vi "AutoDrive PID.vi"(8 "Steady Val (no PID only)":dbl, 9 "Distance to travel (inches)":dbl, 10 "Desired RPM (PID only)":dbl, 11 "Use PID":bool) -> ()   [LabVIEW 2012]
uses:
  State_Machine_Enum.ctl
  Robot Global Data.vi
  <vilib>/addons/control/pid/pid.llb/PID (DBL).vi
  <vilib>/addons/control/pid/NI_PID_pid.lvlib
panel:
  in  "output range LEFT":cluster{"output high":dbl, "output low":dbl}={"output high"=1.0, "output low"=-1.0} {"output low" format="%.2f"; "output high" format="%.2f"}
  in  "Left PID Gains":T1={"proportional gain (Kc)"=0.015, "integral time (Ti, min)"=0.001, "derivative time (Td, min)"=0.0} {"derivative time (Td, min)" format="%.3f"; "integral time (Ti, min)" format="%.3f"; "proportional gain (Kc)" format="%.3f"}
  in  "output range RIGHT":cluster{"output high":dbl, "output low":dbl}={"output high"=1.0, "output low"=-1.0} {"output low" format="%.2f"; "output high" format="%.2f"}
  in  "Right PID Gains":T1={"proportional gain (Kc)"=0.015, "integral time (Ti, min)"=0.001, "derivative time (Td, min)"=0.0} {"derivative time (Td, min)" format="%.3f"; "integral time (Ti, min)" format="%.3f"; "proportional gain (Kc)" format="%.3f"}
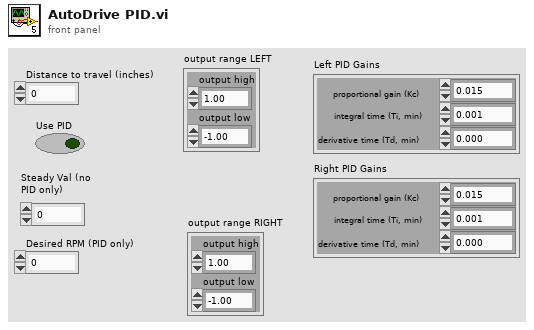
[diagram p1: front panel]
types:
  T1 = cluster{"proportional gain (Kc)":dbl, "integral time (Ti, min)":dbl, "derivative time (Td, min)":dbl}
  T2 = typedef "State_Machine_Enum.ctl" = enum16{"Idle", "Start", "Do", "Stop", "Init"}
  T3 = typedef "LoopDisable.ctl" = cluster{"Climb.vi":bool, "LauncherAngle.vi":bool, "Launcher.vi":bool, "ArmControl.vi":bool, "WinchMotor.vi":bool, "ReadDriveEncoder.vi":bool}
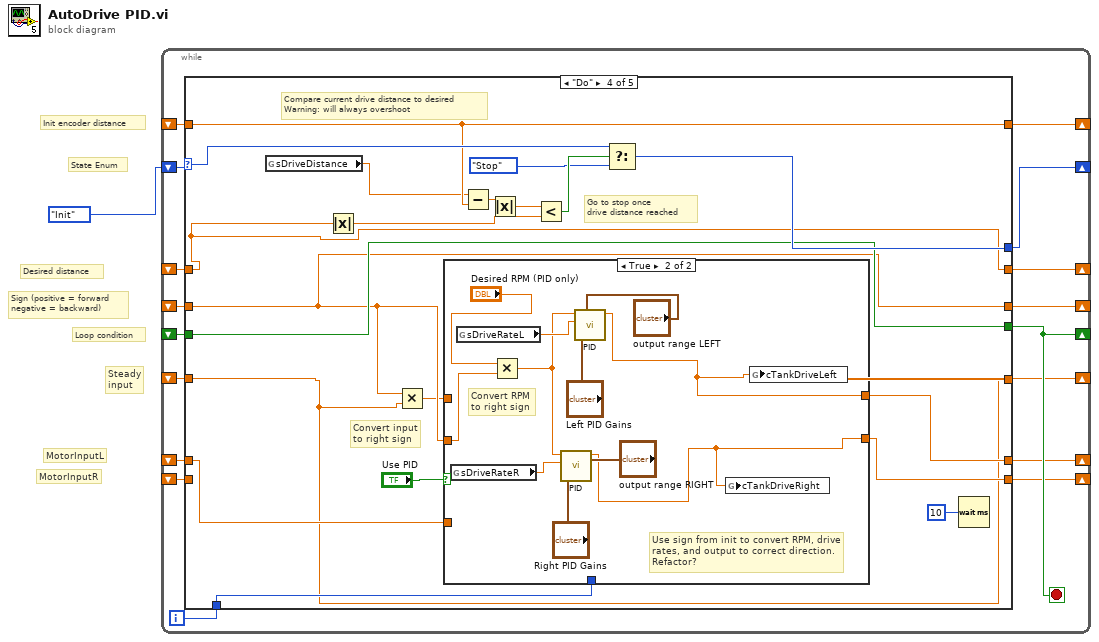
[diagram p0: block diagram]
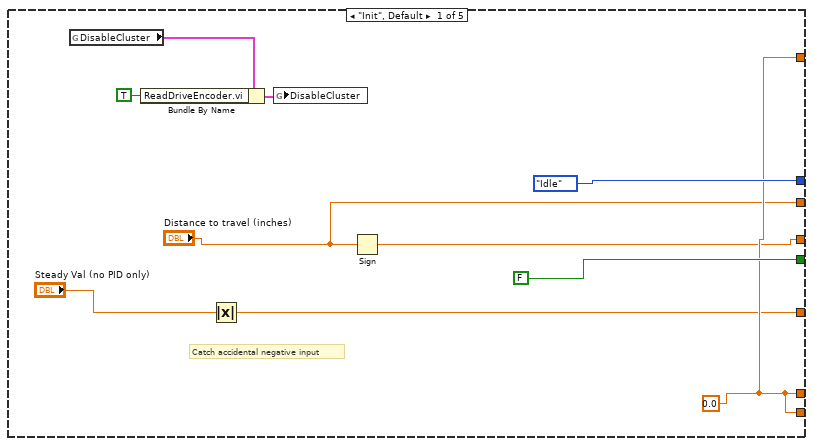
[diagram p2: hidden frame]
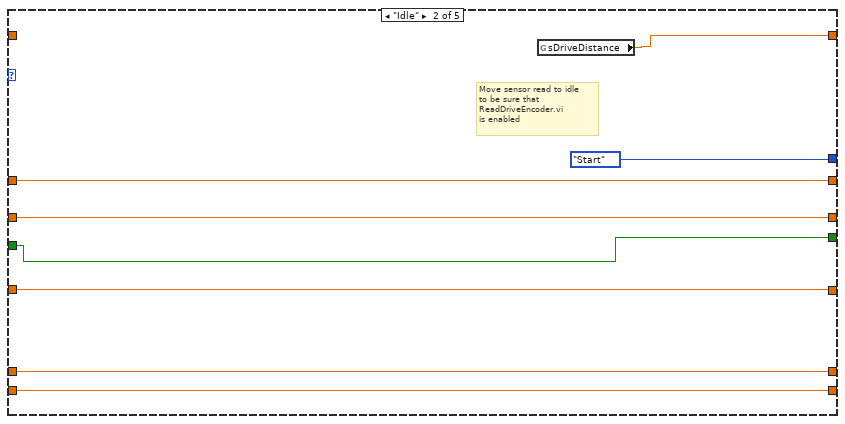
[diagram p3: hidden frame]
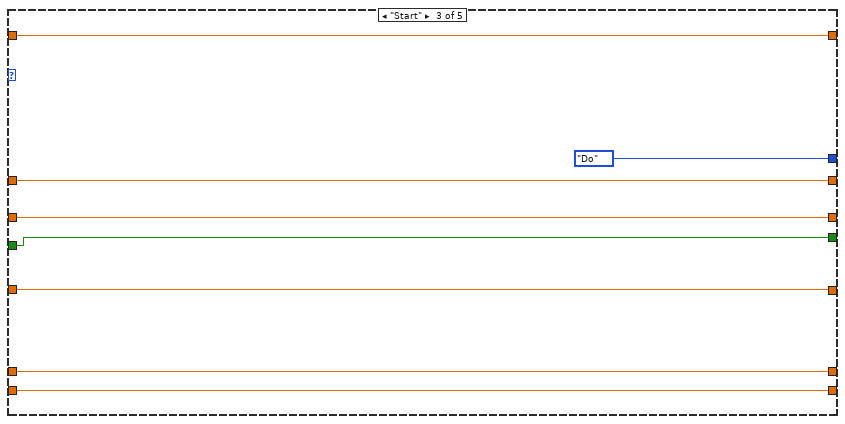
[diagram p4: hidden frame]
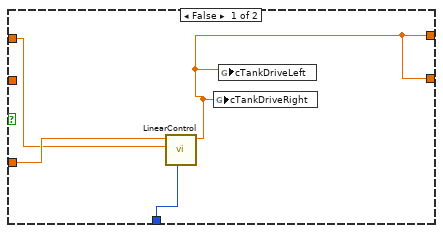
[diagram p5: hidden frame]
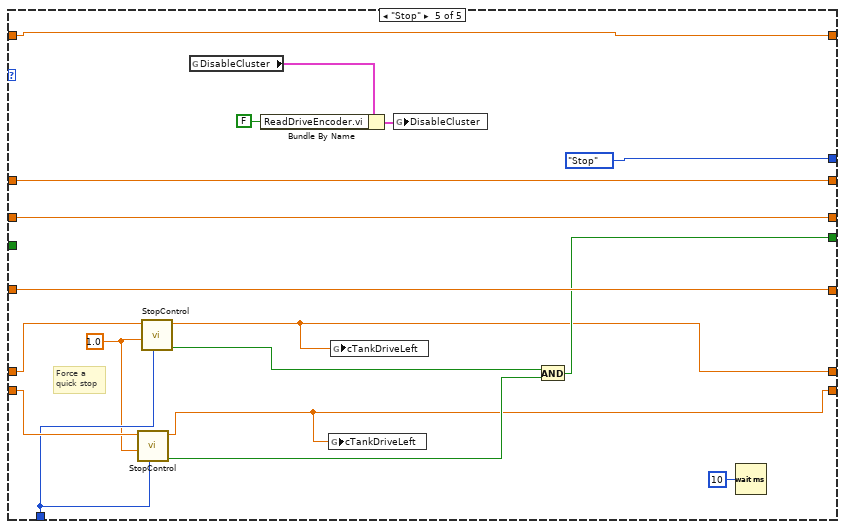
[diagram p6: hidden frame]
diagram:
  # "Desired distance"
  # "MotorInputR"
  # "MotorInputL"
  # "Sign (positive = forward\nnegative = backward)"
  # "Init encoder distance"
  # "State Enum"
  # "Loop condition"
  # "Steady\ninput"
  n1 = while {
    shift-right: [w17] -> _
    shift-left: State_Machine_Enum."Init" ("State") -> [w18]
    shift-right: [w16] -> _
    shift-left: _ -> [w15]
    shift-right: [w14] -> _
    shift-left: _ -> [w13]
    shift-right: [w12] -> _
    shift-left: _ -> [w11]
    shift-right: [w9] -> _
    shift-left: _ -> [w7]
    shift-right: [w10] -> _
    shift-left: _ -> [w8]
    shift-right: [w6] -> _
    shift-left: _ -> [w5]
    shift-right: [w3] -> _
    shift-left: _ -> [w2]
    i -> [w4]
    stop <- w16 stop-if-true
    n2 = case shown="\"Do\"" w18 {
      selector: w18 -> [_ _ _ w64 _]
      tunnel: [State_Machine_Enum."Idle" ("State") State_Machine_Enum."Start" ("State") State_Machine_Enum."Do" ("State") w63 State_Machine_Enum."Stop" ("State")] -> w17
      tunnel: [w19 w32 w40 w46 w88] -> w6
      tunnel: [FALSE w36 w44 w60 w85] -> w16
      tunnel: w15 -> [_ w36 w44 w60 _]
      tunnel: [w23 w31 w43 w58 w97] -> w14
      tunnel: w13 -> [_ _ w43 w58 w97]
      tunnel: [w21 w29 w41 w47 w95] -> w12
      tunnel: w11 -> [_ w29 w41 w47 w95]
      tunnel: [w23 w34 w39 w52 w83] -> w10
      tunnel: [w23 w33 w38 w51 w82] -> w9
      tunnel: w8 -> [_ w34 w39 w50 w90]
      tunnel: w7 -> [_ w33 w38 _ w89]
      tunnel: w5 -> [_ w32 w40 w46 w88]
      tunnel: w4 -> [_ _ _ w49 w81]
      tunnel: ["Distance to travel (inches)" w30 w37 w48 w84] -> w3
      tunnel: w2 -> [_ w30 w37 w48 w84]
      frame "Init", Default {
        w23 = 0.0 ("New Motor Input")
        # "Catch accidental negative input"
        n3 = global read "Robot Global Data.vi" "DisableCluster"() -> (w26:T3)
        n4 = Bundle By Name(cluster=w26, "ReadDriveEncoder.vi"=TRUE) -> (w25:T3)
        n5 = Absolute Value(x="Steady Val (no PID only)") -> (abs(x)=w19:dbl)
        n6 = global write "Robot Global Data.vi" "DisableCluster"(w25) -> ()
        n7 = Sign(1:"Distance to travel (inches)") -> (0:w21:dbl)
      }
      frame "Idle" {
        # "Move sensor read to idle\nto be sure that \nReadDriveEncoder.vi\nis enabled"
        n8 = global read "Robot Global Data.vi" "sDriveDistance"() -> (w31:dbl)
      }
      frame "Start" {
      }
      frame "Do" {
        # "Go to stop once\ndrive distance reached"
        # "Convert input\nto right sign"
        # "Compare current drive distance to desired\nWarning: will always overshoot"
        n9 = global read "Robot Global Data.vi" "sDriveDistance"() -> (w54:dbl)
        n10 = Absolute Value(x=w48) -> (abs(x)=w56:dbl)
        n11 = Multiply(x=w47, y=w46) -> (x*y=w45:dbl)
        n12 = case shown="True" "Use PID" {
          tunnel: w50 -> [w68 _]
          tunnel: w47 -> [_ w72]
          tunnel: [w65 w70] -> w52
          tunnel: [w65 w69] -> w51
          tunnel: w49 -> [w67 _]
          tunnel: w45 -> [w66 _]
          frame False {
            n13 = call "LinearControl.vi"("Loop Iteration"=w67, "Setpoint"=w66, "Motor Value"=w68) -> ("New Motor Value"=w65:dbl)  [unwired: 7 in, 1 out]
            n14 = global write "Robot Global Data.vi" "cTankDriveRight"(w65) -> ()
            n15 = global write "Robot Global Data.vi" "cTankDriveLeft"(w65) -> ()
          }
          frame True {
            # "Convert RPM\nto right sign"
            # "Use sign from init to convert RPM, drive\nrates, and output to correct direction.\nRefactor?"
            n16 = global read "Robot Global Data.vi" "sDriveRateR"() -> (w74:dbl)
            n17 = global read "Robot Global Data.vi" "sDriveRateL"() -> (w75:dbl)
            n18 = Multiply(x="Desired RPM (PID only)", y=w72) -> (x*y=w71:dbl)
            n19 = call-poly <vilib>:"PID.vi"("output range"="output range RIGHT", "PID gains"="Right PID Gains", "process variable"=w74, "setpoint"=w71) -> ("output"=w69:dbl)  [unwired: 6 in, 1 out]
            n20 = call-poly <vilib>:"PID.vi"("output range"="output range LEFT", "PID gains"="Left PID Gains", "process variable"=w75, "setpoint"=w71) -> ("output"=w70:dbl)  [unwired: 6 in, 1 out]
            n21 = global write "Robot Global Data.vi" "cTankDriveRight"(w69) -> ()
            n22 = global write "Robot Global Data.vi" "cTankDriveLeft"(w70) -> ()
          }
        }
        n23 = Subtract(x=w54, y=w58) -> (x-y=w59:dbl)
        n24 = Absolute Value(x=w59) -> (abs(x)=w53:dbl)
        n25 = Less?(x=w53, y=w56) -> (x < y?=w61:bool)
        n26 = Select(t=w64, s=w61, f=State_Machine_Enum."Stop" ("State")) -> (s? t:f=w63:T2)
        n27 = Wait (ms)(milliseconds to wait=u32 10) -> ()  [unwired: 1 out]
      }
      frame "Stop" {
        w80 = 1.0 ("Rate (unit/s)")
        # "Force a\nquick stop"
        n28 = call "StopControl.vi"("Loop Iteration"=w81, "Rate (unit/s)"=w80, "Motor Value"=w89) -> ("Done Stopping"=w86:bool, "New Motor Value"=w82:dbl)  [unwired: 7 in]
        n29 = call "StopControl.vi"("Loop Iteration"=w81, "Rate (unit/s)"=w80, "Motor Value"=w90) -> ("Done Stopping"=w87:bool, "New Motor Value"=w83:dbl)  [unwired: 7 in]
        n30 = global read "Robot Global Data.vi" "DisableCluster"() -> (w94:T3)
        n31 = Bundle By Name(cluster=w94, "ReadDriveEncoder.vi"=FALSE) -> (w93:T3)
        n32 = global write "Robot Global Data.vi" "cTankDriveLeft"(w82) -> ()
        n33 = global write "Robot Global Data.vi" "cTankDriveLeft"(w83) -> ()
        n34 = global write "Robot Global Data.vi" "DisableCluster"(w93) -> ()
        n35 = And(x=w87, y=w86) -> (x .and. y?=w85:bool)
        n36 = Wait (ms)(milliseconds to wait=u32 10) -> ()  [unwired: 1 out]
      }
    }
  }
